vi "Init Stop Notifier.vi"(8 "error in (no error)":errorcluster, 11 "DUT Sample in":refnum<class "DUT Sample.lvclass">) -> (0 "error out":errorcluster, 3 "DUT Sample out":refnum<class "DUT Sample.lvclass">)   [LabVIEW 2023, in "DUT Sample.lvclass"]
uses:
  DUT Sample.lvclass
  DUT Sample.lvclass/DUT Sample.ctl
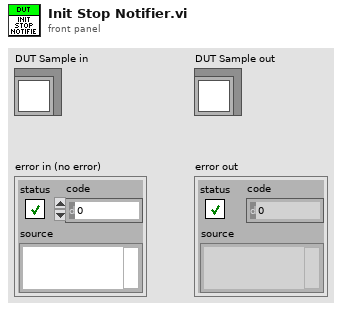
[diagram p1: front panel]
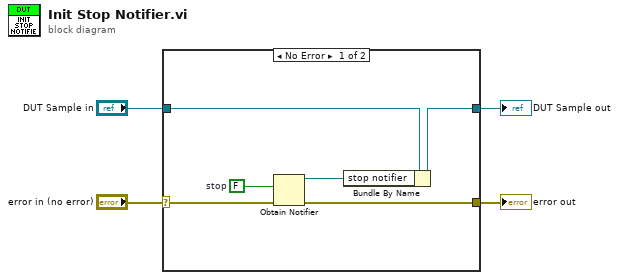
[diagram p0: block diagram]
diagram:
  n1 = case shown="No Error" "error in (no error)" {
    selector: "error in (no error)" -> [w5 w12]
    tunnel: [w6 w12] -> w3
    tunnel: [w8 w11] -> w1
    tunnel: "DUT Sample in" -> [w10 w11]
    frame No Error {
      w9 = FALSE  # stop
      n2 = Obtain Notifier(notification data type=w9, error in (no error)=w5) -> (notifier out=w7:refnum<notifier>, error out=w6:errorcluster)  [unwired: 2 in, 1 out]
      n3 = Bundle By Name(cluster=w10, "stop notifier"=w7) -> (w8:refnum<class "DUT Sample.lvclass">)
    }
    frame Error {
    }
  }
  "error out" <- w3
  "DUT Sample out" <- w1
